vi "Discover Systems.vi"(8 "error in (no error)":errorcluster, 10 "Draw Area Size":T1, 11 "Detected Systems":string[](array[string])) -> (0 "error out":errorcluster, 1 "IP Addresses":string[](array[string]), 2 "Names":string[](array[string]), 3 "RemoteSys Found":refnum<data-value>[](array[refnum]))   [LabVIEW 2016]
uses:
  <vilib>/LIEF/Forms/Shape/Shape.lvclass
  <vilib>/Utility/miscctls.llb/LVBoundsTypeDef.ctl
  Remote System/Remote System.lvclass
  C:/Program Files (x86)/National Instruments/LabVIEW 2016/vi.lib/LIEF/Forms/Shape/Shape.lvclass
  <vilib>/regexp/Match Regular Expression.xnode
  <vilib>/LIEF/Forms/Grid/Grid.lvclass
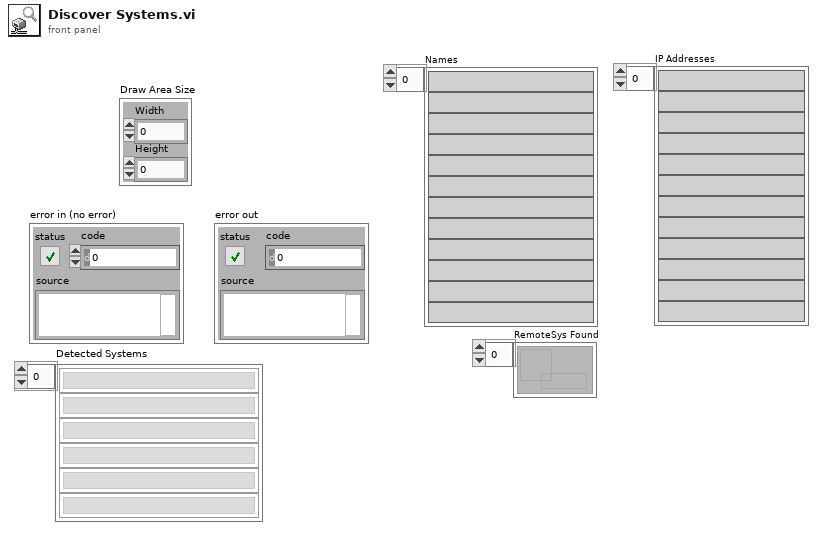
[diagram p1: front panel]
types:
  T1 = typedef "LVBoundsTypeDef.ctl" = cluster{"Width":u32, "Height":u32}
  T2 = enum16{"Left", "Top", "Right", "Bottom", "Centered"}
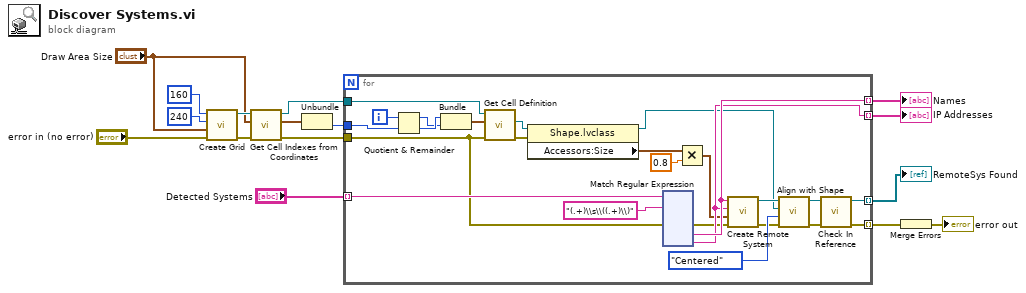
[diagram p0: block diagram]
diagram:
  n1 = call <vilib>:"Create Grid.vi"("error in (no error)"="error in (no error)", "Draw Area"="Draw Area Size", "Horizontal Step"=240, "Vertical Step"=160) -> ("error out"=w3:errorcluster, "Grid Reference"=w5:refnum<data-value>)  [unwired: 6 in]
  n2 = call <vilib>:"Get Cell Indexes from Coordinates.vi"("error in (no error)"=w3, "Coordinates"="Draw Area Size", "Shape Reference"=w5) -> ("error out"=w8:errorcluster, "Indexes"=w11:cluster{"Row":u32, "Column":u32}, "Shape Reference 2"=w9:refnum<data-value>)  [unwired: 6 in]
  n3 = Unbundle(w11) -> ("Column"=w10:u32)  [unwired: 1 out]
  n4 = for {
    tunnel: "Detected Systems" -> [w41] mode=indexing
    tunnel: [w39] -> w16 mode=indexing
    tunnel: [w38] -> w15 mode=indexing
    tunnel: [w36] -> w13 mode=indexing
    tunnel: [w35] -> w12 mode=indexing
    tunnel: w10 -> [w33]
    tunnel: w9 -> [w30]
    tunnel: w8 -> [w17]
    i -> [w34]
    n5 = Quotient & Remainder(x=w34, y=w33) -> (x-y*floor(x/y)=w31:u32, floor(x/y)=w32:u32)
    n6 = Bundle(w32, w31) -> (w29:cluster{u32, u32})  [unwired: 1 in]
    n7 = call <vilib>:"Get Cell Definition.vi"("error in (no error)"=w17, "Indexes"=w29, "Shape Reference"=w30) -> ("error out"=w18:errorcluster, "Cell"=w26:refnum<class "Shape.lvclass">)  [unwired: 6 in, 1 out]
    n8 = property class="Shape.lvclass"(reference=w26, error in=w18) -> (reference out=w22:refnum<class "Shape.lvclass">, "Accessors:Size"=w24:cluster{"Width":i32, "Height":i32})  [unwired: 1 out]
    n9 = xnode "Match Regular Expression"("input string"=w41, "regular expression"="(.+)\\s\\((.+)\\)", "error in"=w17) -> ("error out"=w37:errorcluster, "submatch 1"=w39:string, "submatch 2"=w38:string)  [unwired: 3 in, 4 out]
    n10 = Multiply(x=w24, y=0.8) -> (x*y=w23:cluster{"Width":dbl, "Height":dbl})
    n11 = call "Create Remote System.vi"("error in (no error)"=w37, "Size"=w23, "IP Address"=w38, "System Alias"=w39) -> ("error out"=w20:errorcluster, "Remote System out"=w28:refnum<class "Remote System.lvclass">)  [unwired: 6 in]
    n12 = call <vilib>:"Align with Shape.vi"("error in (no error)"=w20, "Alignment"=T2."Centered", "Reference Shape"=w22, "Shape in"=w28) -> ("error out"=w19:errorcluster, "Shape out"=w21:refnum<class "Remote System.lvclass">)  [unwired: 6 in]
    n13 = call <vilib>:"Check In Reference.vi"("error in (no error)"=w19, "Shape in"=w21) -> ("error out"=w36:errorcluster, "Shape Reference"=w35:refnum<data-value>)  [unwired: 8 in]
  }
  "Names" <- w16
  "IP Addresses" <- w15
  "RemoteSys Found" <- w12
  n14 = Merge Errors(w13) -> (→"error out":errorcluster)
